vi "FlatToRichcif_channelcore_Channels.vi"(5 "OutputClusterType":T1, 11 "InputCluster":T4) -> (3 "OutputCluster":T1)   [LabVIEW 2021, in "CIFCoreChannel_server.lvlib"]
uses:
  CIFCoreChannel_server.lvlib
  cif_channelcore_Channels_Flat.ctl
  cif_channelcore_Channel_Flat.ctl
  cif_channelcore_Direction.ctl
  cif_channelcore_Channels.ctl
  cif_channelcore_Channel.ctl
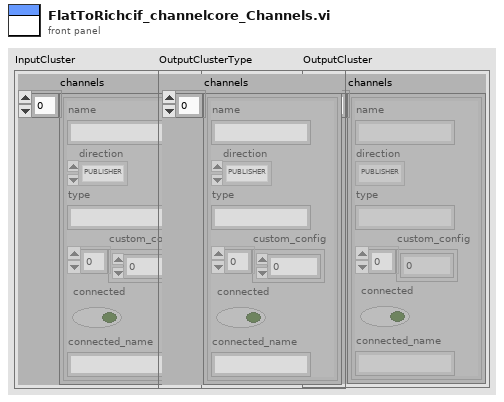
[diagram p1: front panel]
types:
  T1 = typedef "CIFCoreChannel_server.lvlib/cif_channelcore_Channels.ctl" = cluster{"channels":T2[]}
  T2 = typedef "CIFCoreChannel_server.lvlib/cif_channelcore_Channel.ctl" = cluster{"name":string, "direction":T3, "type":string, "custom_config":u8[], "connected":bool, "connected_name":string}
  T3 = typedef "CIFCoreChannel_server.lvlib/cif_channelcore_Direction.ctl" = enum32{"PUBLISHER", "SUBSCRIBER"}
  T4 = typedef "CIFCoreChannel_server.lvlib/cif_channelcore_Channels_Flat.ctl" = cluster{"channels":T5[]}
  T5 = typedef "CIFCoreChannel_server.lvlib/cif_channelcore_Channel_Flat.ctl" = cluster{"name":string, "direction":T3, "type":string, "custom_config":u8[], "connected":bool, "connected_name":string}
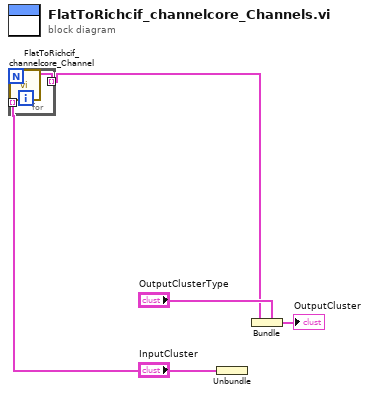
[diagram p0: block diagram]
diagram:
  n1 = Unbundle "Unbundle"("InputCluster") -> ("channels"=w2:T5[])
  n2 = for {
    tunnel: w2 -> [w7] mode=indexing
    tunnel: [w6] -> w1 mode=indexing
    n3 = call "FlatToRichcif_channelcore_Channel.vi"("InputCluster"=w7) -> ("OutputCluster"=w6:T2)  [unwired: 10 in]
  }
  n4 = Bundle "Bundle"(cluster="OutputClusterType", "channels"=w1) -> (→"OutputCluster":T1)
